vi "ResonanceAnalyzer.vi"() -> ()   [LabVIEW 2015]
uses:
  <vilib>/imath/engines/lvmath2/RunTimeEngine/Managers/WorkSpace/UID Generator.vi
  <vilib>/imath/engines/lvmath2/RunTimeEngine/RunTimeType/NIMS_RunTimeType_From StrictType (excl LVString).vi
  <instcachedir>/0/NIMS_RunTimeType_From StrictType (excl LVString)_EB1C38A9BC5048DA9ABDA8F781E54D21.lvgen/NIMS_RunTimeType_From StrictType (excl LVString)_EB1C38A9BC5048DA9ABDA8F781E54D21_000.vi
  <vilib>/imath/engines/lvmath2/RunTimeEngine/LocalVariableDefStatement/MC_LocalVariableDefStatement_Display.vi
  <vilib>/imath/engines/lvmath2/RunTimeEngine/RangeToken/NIMS_Range.vi
  <instcachedir>/0/NIMS_Range_D919CC09935940E88F755EC1C6F49AC1.lvgen/NIMS_Range_D919CC09935940E88F755EC1C6F49AC1_000.vi
  <vilib>/imathl/engines/lvmath/Functions/Error Handling/Create Error.vi
  <vilib>/imath/engines/lvmath2/RunTimeEngine/BuiltInFunctions/randnormal/NIMS_randnormal(1,I32).vi
  <vilib>/imath/engines/lvmath2/RunTimeEngine/ErrorHandling/NIMS_Error From Error Code.vi
  <vilib>/imath/engines/lvmath2/RunTimeEngine/ArithmeticOperatorToken/NIMS_ArithmeticOperator_plus.vi
  <instcachedir>/0/NIMS_ArithmeticOperator_plus_A4F2756F5ADB4A0090E0DBD7C10701C8.lvgen/NIMS_ArithmeticOperator_plus_A4F2756F5ADB4A0090E0DBD7C10701C8_004.vi
  <vilib>/imath/engines/lvmath2/RunTimeEngine/Managers/SymbolTable/Clear UID.vi
  <vilib>/imath/engines/lvmath2/RunTimeEngine/NodeEndStatement/NIMS_NodeEndStatement_Output.vi
  <instcachedir>/0/NIMS_NodeEndStatement_Output_53EC0D466D134D7ABD903AC30B43404B.lvgen/NIMS_NodeEndStatement_Output_53EC0D466D134D7ABD903AC30B43404B_005.vi
  <vilib>/imath/engines/lvmath2/RunTimeEngine/ErrorHandling/NIMS_Finalize Error.vi
  <vilib>/Utility/file.llb/Read Delimited Spreadsheet (DBL).vi
  <vilib>/imath/engines/lvmath2/RunTimeEngine/Managers/SymbolTable/NIMS_WorkSpace.lvlib
panel:
  out "Array":dbl[](array[numeric])
  out "XY Graph":cluster{"all rows":dbl[], "Array":dbl[]}[](graph)
  in  "Tab Control":enum32{"Simulation", "Experiment"}(tab)
  in  "Q":dbl
  in  "Center Frequency":dbl
  in  "Start Frequency":dbl
  in  "End Frequency":dbl
  in  "df":dbl
  in  "Noise Level":dbl
  in  "file path (dialog if empty)":path
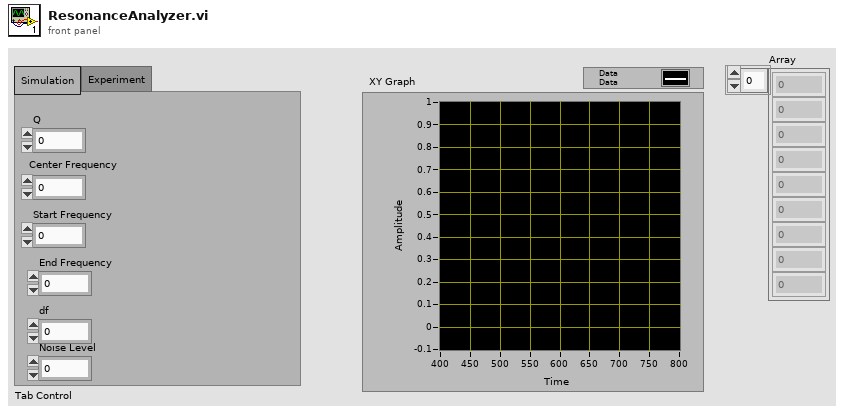
[diagram p1: front panel]
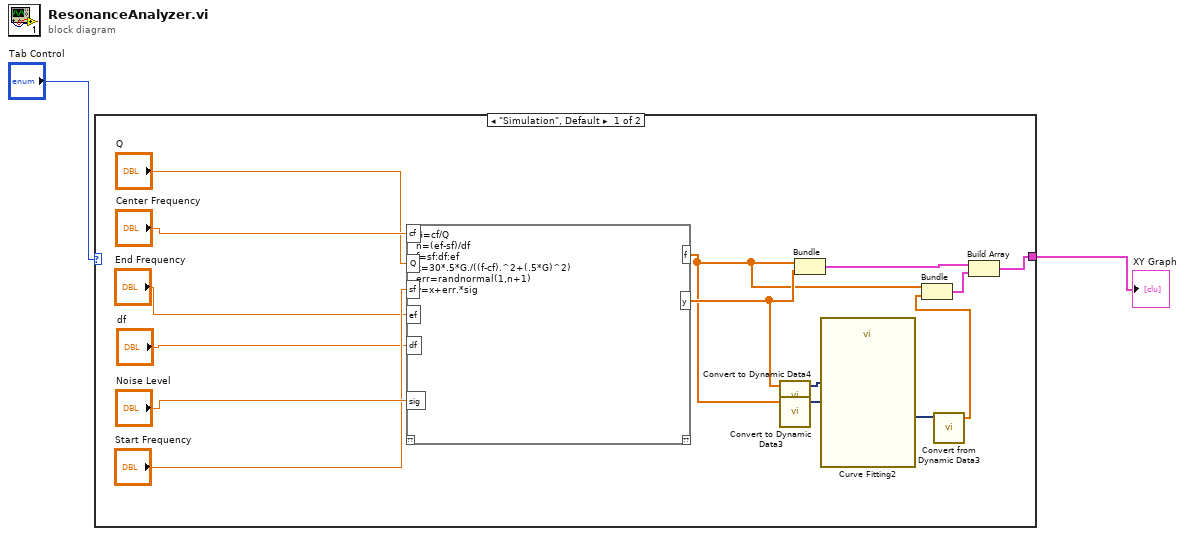
[diagram p0: block diagram]
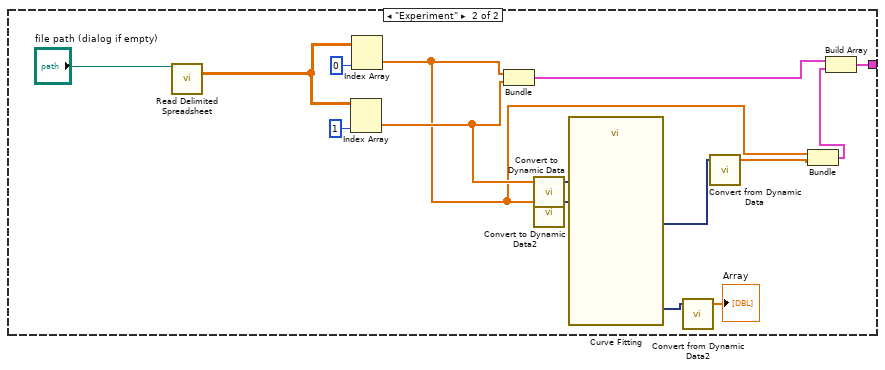
[diagram p2: hidden frame]
diagram:
  n1 = case shown="\"Simulation\", Default" "Tab Control" {
    tunnel: [w8 w194] -> w1
    frame "Simulation", Default {
      n2 = mathscript code="G=cf/Q\nn=(ef-sf)/df\nf=sf:df:ef\nx=30*.5*G./((f-cf).^2+(.5*G)^2)\nerr=randnormal(1,n+1)\ny=x+err.*sig"("sig"="Noise Level", "cf"="Center Frequency", "sf"="Start Frequency", "ef"="End Frequency", "df"="df", "Q"="Q") -> ("y"=w11:dbl[], "f"=w6:dbl[])  [unwired: 1 in, 1 out]
      n3 = call "Convert to Dynamic Data4"("Array"=w11) -> ("Dynamic Data Type"=w5:dynamicdata)  [unwired: 3 in]
      n4 = call "Convert to Dynamic Data3"("Array"=w6) -> ("Dynamic Data Type"=w4:dynamicdata)  [unwired: 3 in]
      n5 = Bundle("f"=w6, "y"=w11) -> (w10:cluster{"f":dbl[], "y":dbl[]})  [unwired: 1 in]
      n6 = call "Curve Fitting2"("Locations"=w4, "Signals"=w5) -> ("best fit"=w3:dynamicdata)  [unwired: 6 in, 3 out]
      n7 = call "Convert from Dynamic Data3"("Dynamic Data Type"=w3) -> ("Array"=w7:dbl[])  [unwired: 3 in]
      n8 = Bundle("f"=w6, "Array"=w7) -> (w9:cluster{"f":dbl[], "Array":dbl[]})  [unwired: 1 in]
      n9 = Build Array(w10, w9) -> (w8:cluster{"f":dbl[], "Array":dbl[]}[])
    }
    frame "Experiment" {
      n10 = call-poly <vilib>:"Read Delimited Spreadsheet.vi"("file path (dialog if empty)"="file path (dialog if empty)") -> ("all rows"=w205:dbl[][])  [unwired: 9 in, 5 out]
      n11 = Index Array(array=w205, index (col)=1 ("disabled index (col)")) -> (element=w202:dbl[])  [unwired: 1 in]
      n12 = Index Array(array=w205, index (col)=0 ("disabled index (col)")) -> (element=w197:dbl[])  [unwired: 1 in]
      n13 = Bundle("all rows"=w197, "all rows"=w202) -> (w196:cluster{"all rows":dbl[], "all rows":dbl[]})  [unwired: 1 in]
      n14 = call "Convert to Dynamic Data"("Array"=w202) -> ("Dynamic Data Type"=w201:dynamicdata)  [unwired: 3 in]
      n15 = call "Convert to Dynamic Data2"("Array"=w197) -> ("Dynamic Data Type"=w200:dynamicdata)  [unwired: 3 in]
      n16 = call "Curve Fitting"("Locations"=w200, "Signals"=w201) -> ("best fit"=w199:dynamicdata, "non-linear coefficients"=w193:dynamicdata)  [unwired: 5 in, 3 out]
      n17 = call "Convert from Dynamic Data2"("Dynamic Data Type"=w193) -> ("Array"=→"Array":dbl[])  [unwired: 3 in]
      n18 = call "Convert from Dynamic Data"("Dynamic Data Type"=w199) -> ("Array"=w198:dbl[])  [unwired: 3 in]
      n19 = Bundle("all rows"=w197, "Array"=w198) -> (w195:cluster{"all rows":dbl[], "Array":dbl[]})  [unwired: 1 in]
      n20 = Build Array(w196, w195) -> (w194:cluster{"all rows":dbl[], "Array":dbl[]}[])
    }
  }
  "XY Graph" <- w1
